vi "Dynamic Signal Analyzer (sim).vi"() -> ()   [LabVIEW 2023]
doc: "Simulates a general purpose Dynamic Signal Analyzer using the Waveform Measurement and Generation VIs. The example's functionality includes single and two-channel signal processing such as power spectrum, frequency response, coherence and so on, windowing, averaging, and conversion to typical display units. You can easily customize this example."
panel:
  in  "Stop":bool
  in  "view":cluster{"Channel":u16, "View 2":u16} {"View 2" items=["Magnitude", "Phase", "Coherence (FRF only)"]; "Channel" items=["Channel A (stimulus)", "Channel B (Response)"]}
  in  "DSA settings":T1={"function"=enum."Frequency response", "baseband span"=20000.0, "window"=enum."Hanning", "resolution (# of lines)"=800} {"baseband span" format="%#.6g"}
  in  "signal generator":T2={"Waveform"=enum."Uniform White noise", "frequency"=200.0, "amplitude"=1.0} {"amplitude" format="%#.6g"; "frequency" format="%#.6g"}
  in  "restart averaging":bool
  in  "averaging parameters":T3={"averaging mode"=enum."RMS averaging", "weighting mode"=enum."Exponential", "number of averages"=10} {"number of averages" min=1}
  out "spectral domain":cluster{"f0":dbl, "df":dbl, dbl[]}(graph)
  out "time domain":waveform(dbl)[](graph)
  # "Overview: This VI simulates a general purpose Dynamic Signal Analyzer.\nRequirements: LabVIEW Full Development System\nInstructions: \n1. Run the VI.\n2. Change the DSA settings function value to explore various single and dual-channel measurements.  The single-channel functions are Windowed time, FFT, and Power Spectrum.  Use the view control to select which single-channel to display in the spectral domain.\n3. Click Stop to stop the VI."
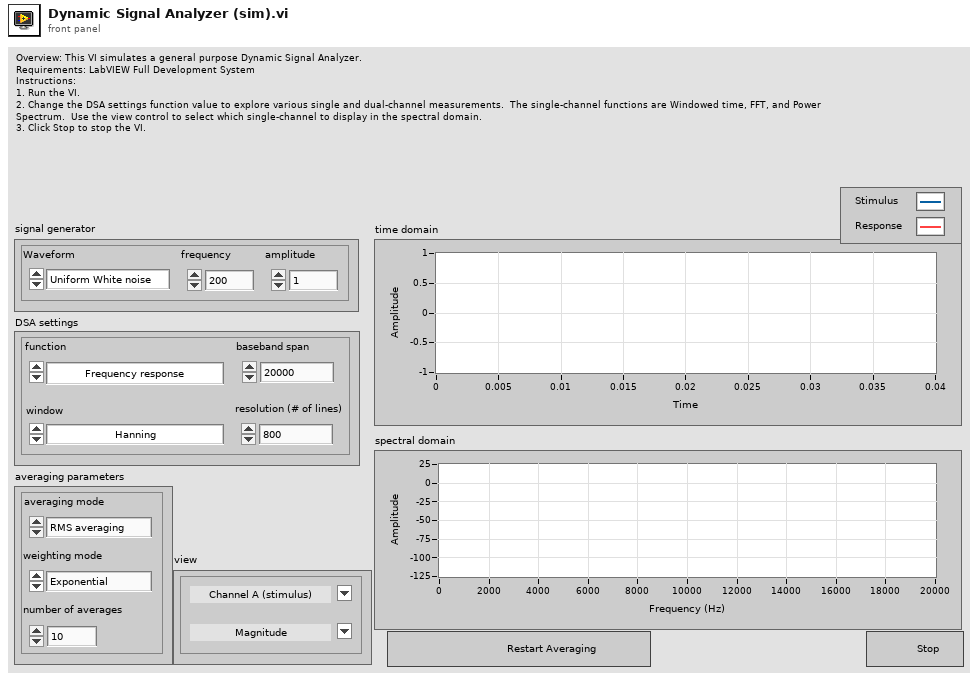
[diagram p1: front panel]
types:
  T1 = cluster{"function":enum16{"Windowed time", "Power Spectrum", "FFT (Mag-Phase)", "Cross Power spectrum", "Frequency response"}, "baseband span":dbl, "window":enum16{"None ", "Hanning", "Hamming", "Blackman-Harris", "Exact Blackman", "Blackman", "Flat Top", "4 Term B-Harris ", "7 Term B-Harris", "Low Sidelobe"}, "resolution (# of lines)":u32}
  T2 = cluster{"Waveform":enum16{"Sine", "Square", "Triangle", "Sawtooth", "Chirp", "Uniform White noise", "Gaussian white noise", "PRN"}, "frequency":dbl, "amplitude":dbl}
  T3 = cluster{"averaging mode":enum16{"No averaging", "Vector averaging", "RMS averaging", "Peak hold"}, "weighting mode":enum16{"Linear", "Exponential"}, "number of averages":u32}
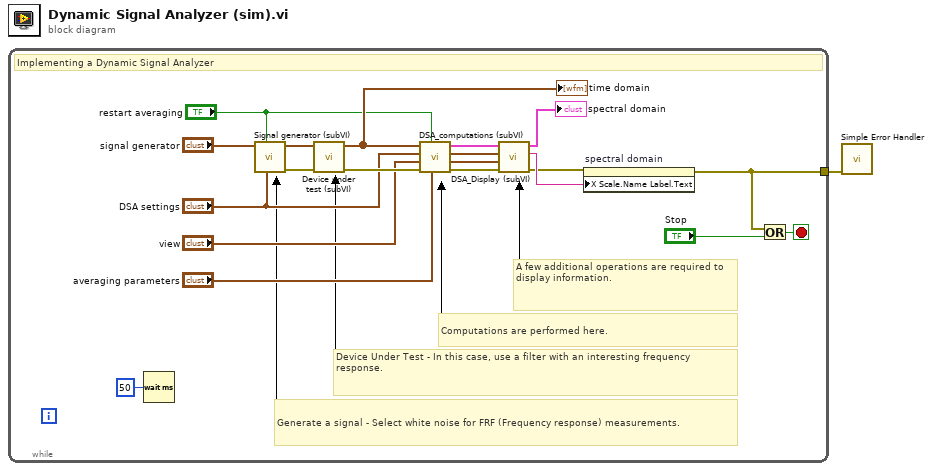
[diagram p0: block diagram]
diagram:
  n1 = while {
    tunnel: [w3] -> w1
    stop <- w8 stop-if-true
    # "A few additional operations are required to display information."
    # "Computations are performed here."
    # "Device Under Test - In this case, use a filter with an interesting frequency response."
    # "Generate a signal - Select white noise for FRF (Frequency response) measurements."
    # "Implementing a Dynamic Signal Analyzer"
    n2 = Wait (ms)(milliseconds to wait=u32 50) -> ()  [unwired: 1 out]
    n3 = call "Signal generator (subVI).vi"("DSA settings"="DSA settings", "reset signal"="restart averaging", "signal generator"="signal generator") -> ("error out"=w19:errorcluster, "signal out"=w20:waveform(dbl))  [unwired: 7 in]
    n4 = call "Device under test (subVI).vi"("error in (no error)"=w19, "signal in"=w20) -> ("error out"=w21:errorcluster, "stimulus and response"=w10:waveform(dbl)[])  [unwired: 8 in]
    "time domain" <- w10
    n5 = call "DSA_computations (subVI).vi"("averaging parameters"="averaging parameters", "Restart Averaging"="restart averaging", "error in (no error)"=w21, "view"="view", "DSA settings"="DSA settings", "stimulus and response"=w10) -> ("error out"=w16:errorcluster, "view out"=w12:cluster{"Channel":u16, "View":u16}, "DSA settings out"=w7:T1, "output array"=w17:cluster{"f0":dbl, "df":dbl, "Y":dbl[]}[])  [unwired: 2 in]
    n6 = call "DSA_Display (subVI).vi"("error in (no error)"=w16, "view"=w12, "DSA settings"=w7, "stimulus and response"=w17) -> ("error out"=w4:errorcluster, "X Units"=w11:string, "selected display"=→"spectral domain":cluster{"f0":dbl, "df":dbl, "Y":dbl[]})  [unwired: 5 in]
    n7 = property on="spectral domain" class="WFGraph (strict)"(error in=w4, "X Scale.Name Label.Text"=w11) -> (error out=w3:errorcluster)  [unwired: 1 in, 1 out]
    n8 = Or(x=w3, y="Stop") -> (x .or. y?=w8:bool)
  }
  n9 = call <vilib>:"Simple Error Handler.vi"("error in (no error)"=w1) -> ()  [unwired: 4 in, 5 out]
